vi "Update.NSteps.vi"(11 "DyeLaser In":T1={"Scan.Start (cm-1)"=15000.0, "Scan.Stop (cm-1)"=15050.0, "Scan.step (cm-1)"=0.2, "dye laser port"="", "Laser"=enum."Syrah", "NPoints"=251, "CurrentStep"=75, "Current.cm-1"=15015.0} {"Current.cm-1" format="%.2f"}) -> (3 "DyeLaser out":T1={"Scan.Start (cm-1)"=15000.0, "Scan.Stop (cm-1)"=15050.0, "Scan.step (cm-1)"=0.2, "dye laser port"="", "Laser"=enum."Syrah", "NPoints"=251, "CurrentStep"=75, "Current.cm-1"=15015.0} {"Current.cm-1" format="%.2f"})   [LabVIEW 2022 SP3]
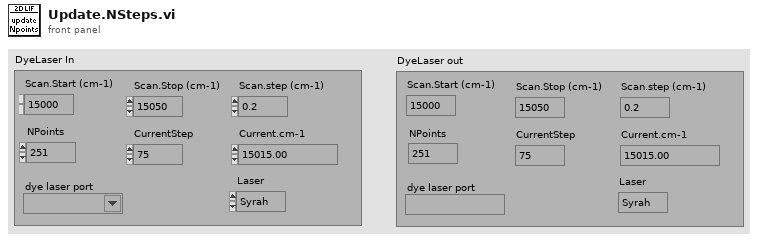
[diagram p1: front panel]
types:
  T1 = cluster{"Scan.Start (cm-1)":dbl, "Scan.Stop (cm-1)":dbl, "Scan.step (cm-1)":dbl, "dye laser port":refnum<visa-resource-name>, "Laser":enum16{"Syrah", "Hyperdye"}, "NPoints":i32, "CurrentStep":i32, "Current.cm-1":dbl}
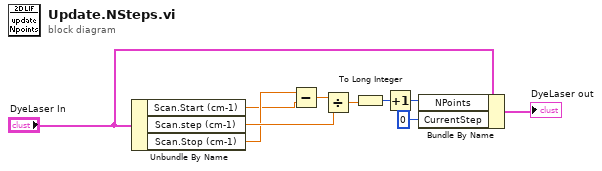
[diagram p0: block diagram]
diagram:
  n1 = Unbundle By Name("DyeLaser In") -> ("Scan.Start (cm-1)"=w5:dbl, "Scan.step (cm-1)"=w8:dbl, "Scan.Stop (cm-1)"=w6:dbl)
  n2 = Subtract(x=w6, y=w5) -> (x-y=w7:dbl)
  n3 = Divide(x=w7, y=w8) -> (x/y=w9:dbl)
  n4 = To Long Integer(number=w9) -> (32bit integer=w10:i32)
  n5 = Increment(x=w10) -> (x+1=w3:i32)
  n6 = Bundle By Name(cluster="DyeLaser In", "NPoints"=w3, "CurrentStep"=0) -> (→"DyeLaser out":T1)
